vi "sv_Get TDMS Feature Group Name String.vi"(7 "feature":T2=1 items=["Features", "RMS Level", "Peak Level", "Max-Min Level", "Band_", "Frequency", "SpectrumFrequency_", "SpectrumAmplitude_", "SpectrumPhase_", "Speed", "Order_", "OrderMagnitude_", "OrderPhase_"]) -> (6 "feature group name":string, 8 "timestamp group name":string, 10 "alarm group names":T1)   [LabVIEW 2017]
uses:
  <vilib>/addons/_NISVFA/_Shared subVIs/Controls/NI Dynamic Features.ctl
  <vilib>/regexp/Match Regular Expression.xnode
panel:
  in  "index":i32
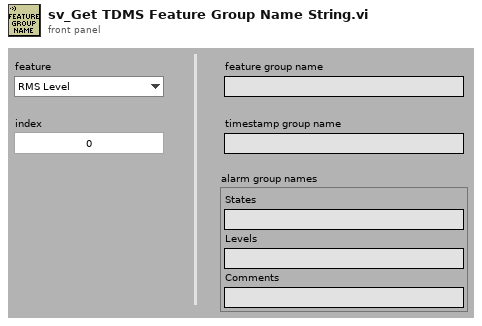
[diagram p1: front panel]
types:
  T1 = cluster{"States":string, "Levels":string, "Comments":string}
  T2 = typedef "NI Dynamic Features.ctl" = u16
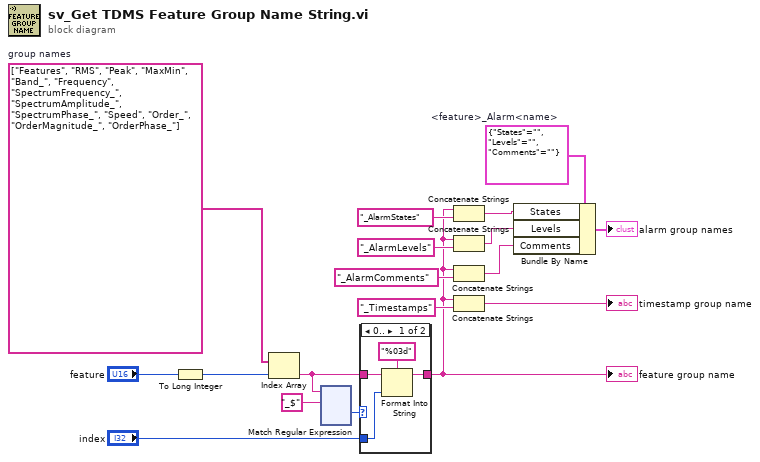
[diagram p0: block diagram]
diagram:
  w4 = T1 {"States"="", "Levels"="", "Comments"=""}  # <feature>_Alarm<name>
  w14 = string[] ["Features", "RMS", "Peak", "MaxMin", "Band_", "Frequency", "SpectrumFrequency_", "SpectrumAmplitude_", "SpectrumPhase_", "Speed", "Order_", "OrderMagnitude_", "OrderPhase_"]  # group names
  n1 = To Long Integer(number="feature") -> (32bit integer=w12:i32)
  n2 = Index Array(array=w14, index=w12) -> (element=w8:string)
  n3 = xnode "Match Regular Expression"("input string"=w8, "regular expression"="_$") -> ("offset past match"=w10:i32)  [unwired: 4 in, 4 out]
  n4 = case shown="0.." w10 {
    tunnel: w8 -> [w20 w23]
    tunnel: [w19 w23] -> w9
    tunnel: "index" -> [w21 _]
    frame 0.. {
      n5 = Format Into String(format string="%03d", initial string=w20, w21) -> (resulting string=w19:string)  [unwired: 1 in, 1 out]
    }
    frame -1, Default {
    }
  }
  "feature group name" <- w9
  n6 = Concatenate Strings(w9, "_AlarmStates" ("string")) -> (w7:string)
  n7 = Concatenate Strings(w9, "_AlarmLevels" ("string")) -> (w6:string)
  n8 = Concatenate Strings(w9, "_AlarmComments" ("string")) -> (w5:string)
  n9 = Concatenate Strings(w9, "_Timestamps" ("string")) -> (→"timestamp group name":string)
  n10 = Bundle By Name(cluster=w4, "States"=w7, "Levels"=w6, "Comments"=w5) -> (→"alarm group names":T1)
